vi "Provision RT Target.vi"() -> ()   [LabVIEW 2020]
uses:
  <vilib>/nisyscfg/Firmware Status.ctl
  <vilib>/nisyscfg/Software 1.2.ctl
  <vilib>/nisyscfg/Component Type.ctl
  <vilib>/nisyscfg/Network Settings Format.ctl
  <vilib>/nisyscfg/Upgrade Firmware (File).vi
  <vilib>/nisyscfg/Close (Hardware).vi
  <vilib>/nisyscfg/Format With Base System Image.vi
  <vilib>/nisyscfg/Close (System).vi
  <vilib>/nisyscfg/nisyscfg.lvlib
  <resource>/objmgr/nisysapi.rc
panel:
  out "New Firmware Revision":string
  out "Real-Time:System Status":string
  in  "Base System Image":T1={"title"="Linux RT System Image 20.5", "description"="", "ID"="{3CDECBF0-04E7-462E-BDD2-2AD4D9B02235}", "version"="20.5.0", "component type"=2} caption="software" {"component type" items=["standard", "hidden", "system", "unknown", "startup", "image", "essential"]}
  in  "Firmware File":path=path "C:/Program Files (x86)/National Instruments/Shared/Firmware/cRIO/76D6/cRIO-9068_8.5.0.cfg"
  out "Detailed Result":string
  out "Firmware Status":T3=2 items=["update pending auto restart"=-4, "verifying new image"=-3, "writing/flashing new image"=-2, "waiting for image"=-1, "corrupt firmware, cannot run"=0, "no firmware installed"=1, ""=2, "update pending user restart"=3, "update pending user action"=4, "update attempt failed"=5]
  out "Current Firmware Revision":string
  out "error out":errorcluster
  in  "Session in":refnum<k21>="Josh-9068 (10.2.67.29)"
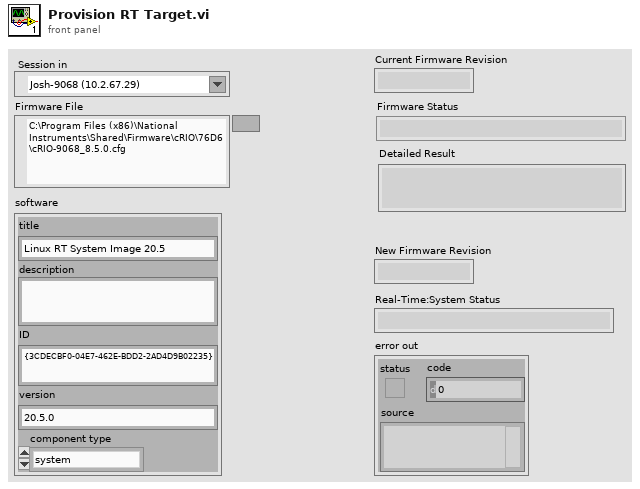
[diagram p1: front panel]
types:
  T1 = typedef "nisyscfg.lvlib/Software 1.2.ctl" = cluster{"title":string, "description":string, "ID":string, "version":string, "component type":T2}
  T2 = typedef "nisyscfg.lvlib/Component Type.ctl" = u32
  T3 = typedef "nisyscfg.lvlib/Firmware Status.ctl" = i32
  T4 = typedef "nisyscfg.lvlib/Network Settings Format.ctl" = u32
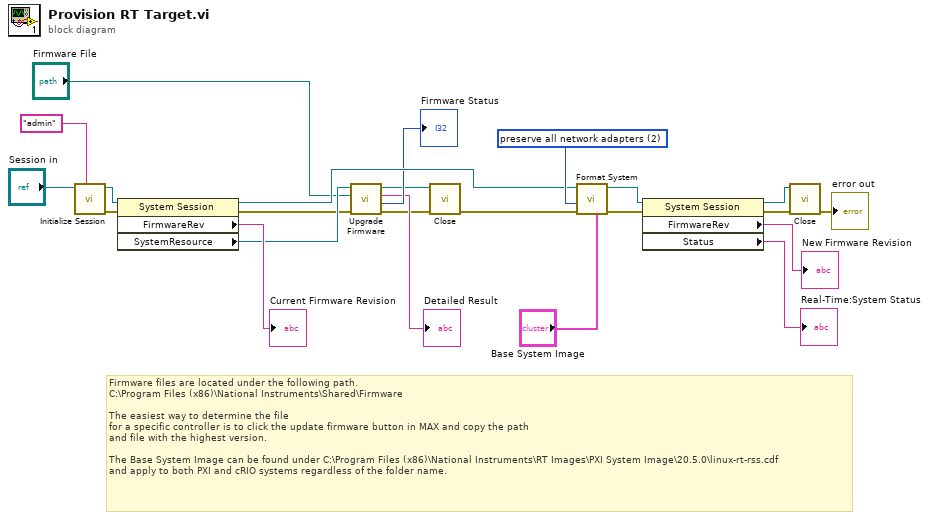
[diagram p0: block diagram]
diagram:
  w23 = T4 2 items=["reset all network adapters", "preserve primary, reset others", "preserve all network adapters"] ("Network Settings (reset all adapters)")
  # "Firmware files are located under the following path. \nC:\\Program Files (x86)\\National Instruments\\Shared\\Firmware\n\nThe easiest way to determine the file\nfor a specific controller is to click the update firmware button in MAX and copy the path \nand file with the highest version.\n\nThe Base System Image can be found under C:\\Program Files (x86)\\National Instruments\\RT Images\\PXI System Image\\20.5.0\\linux-rt-rss.cdf\nand apply to both PXI and cRIO systems regardless of the folder name."
  n1 = call <vilib>:"Initialize Session.vi"("User Name"="admin", "Target (localhost)"="Session in") -> ("error out"=w12:errorcluster, "Session out"=w13:refnum<k21>)  [unwired: 8 in]
  n2 = property class="System Session"(reference=w13, error in=w12) -> (reference out=w21:refnum<k21>, error out=w15:errorcluster, "FirmwareRev"=→"Current Firmware Revision":string, "SystemResource"=w19:refnum<k20>)
  n3 = call-poly <vilib>:"Upgrade Firmware.vi"("error in (no error)"=w15, "Firmware File"="Firmware File", "Resource in"=w19) -> ("error out"=w8:errorcluster, "Firmware Status"=→"Firmware Status":T3, "Detailed Result"=→"Detailed Result":string, "Resource out"=w6:refnum<k20>)  [unwired: 5 in]
  n4 = call-poly <vilib>:"Close.vi"("error in (no error)"=w8, "Resource in"=w6) -> ("error out"=w7:errorcluster)  [unwired: 9 in]
  n5 = call-poly <vilib>:"Format System.vi"("Base System Image"="Base System Image", "error in (no error)"=w7, "Network Settings (reset all adapters)"=w23, "Session in"=w21) -> ("error out"=w9:errorcluster, "Session out"=w10:refnum<k21>)  [unwired: 6 in]
  n6 = property class="System Session"(reference=w10, error in=w9) -> (reference out=w3:refnum<k21>, error out=w5:errorcluster, "FirmwareRev"=→"New Firmware Revision":string, "Status"=→"Real-Time:System Status":string)
  n7 = call-poly <vilib>:"Close.vi"("error in (no error)"=w5, "Session in"=w3) -> ("error out"=→"error out":errorcluster)  [unwired: 9 in]
